vi "Time out.vi"(8 "error in (no error)":errorcluster, 10 "New Time":u32, 11 "Channel GUI in":refnum<class "Channel.lvclass">) -> (0 "error out":errorcluster, 2 "time out ?":bool, 3 "Channel GUI out":refnum<class "Channel.lvclass">)   [LabVIEW 2018, in "Channel.lvclass"]
uses:
  Channel.lvclass
  Channel.lvclass/Channel.ctl
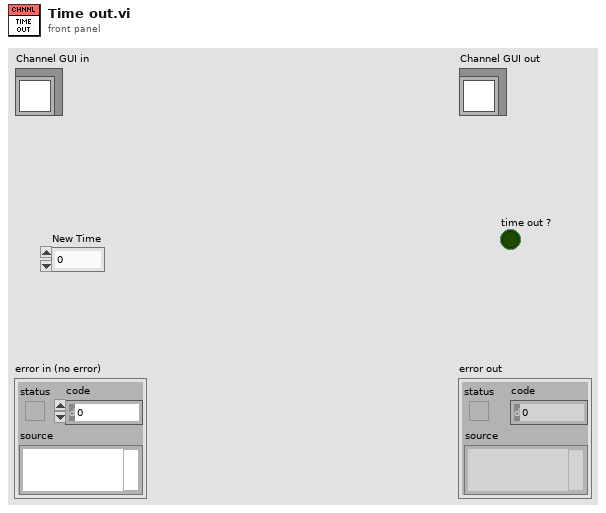
[diagram p1: front panel]
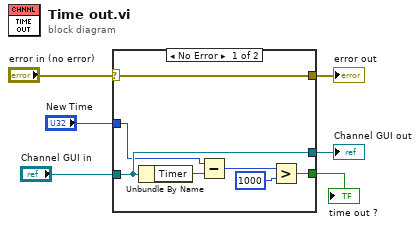
[diagram p0: block diagram]
diagram:
  n1 = case shown="No Error" "error in (no error)" {
    selector: "error in (no error)" -> [w13 w15]
    tunnel: [w13 w15] -> w5
    tunnel: [w12 w14] -> w4
    tunnel: "Channel GUI in" -> [w12 w14]
    tunnel: "New Time" -> [w11 _]
    tunnel: [w7 _] -> w1
    frame No Error {
      n2 = Unbundle By Name(w12) -> ("Timer"=w10:u32)
      n3 = Subtract(x=w11, y=w10) -> (x-y=w9:u32)
      n4 = Greater?(x=w9, y=u32 1000) -> (0:w7:bool)
    }
    frame Error {
    }
  }
  "error out" <- w5
  "Channel GUI out" <- w4
  "time out ?" <- w1
